vi "AttackerBallOutOfFieldSkill.vi"(6 "DistanceToBallOut":i32, 8 "error in (no error)":errorcluster, 9 "Game":refnum<class "Game.lvclass">, 10 "Robot":refnum<class "Robot.lvclass">, 11 "AttackerBallOutOfFieldSkill in":refnum<class "AttackerBallOutOfFieldSkill.lvclass">) -> (0 "error out":errorcluster, 2 "Robot out":refnum<class "Robot.lvclass">, 3 "AttackerBallOutOfFieldSkill out":refnum<class "AttackerBallOutOfFieldSkill.lvclass">)   [LabVIEW 2018, in "AttackerBallOutOfFieldSkill.lvclass"]
uses:
  AttackerBallOutOfFieldSkill.lvclass
  Game_class/Game.lvclass
  Robot_class/Robot.lvclass
  C:/Users/Gustavo/Desktop/RoboIME/SimplePass/SSL_AI/Object_class/Object.lvclass
  Object_class/Object.lvclass/Object.ctl
  Game_class/Game.lvclass/Game.ctl
  Robot_class/Robot.lvclass/Robot.ctl
  Game_class/Read BallRef.vi
  Game_class/Read FieldRef.vi
  Object_class/Read x.vi
  Object_class/Read y.vi
  Robot_class/Write dest_x.vi
  Robot_class/Write dest_y.vi
  Robot_class/Write dest_orientation.vi
  Ball_class/Ball.lvclass
  Field_class/Field.lvclass
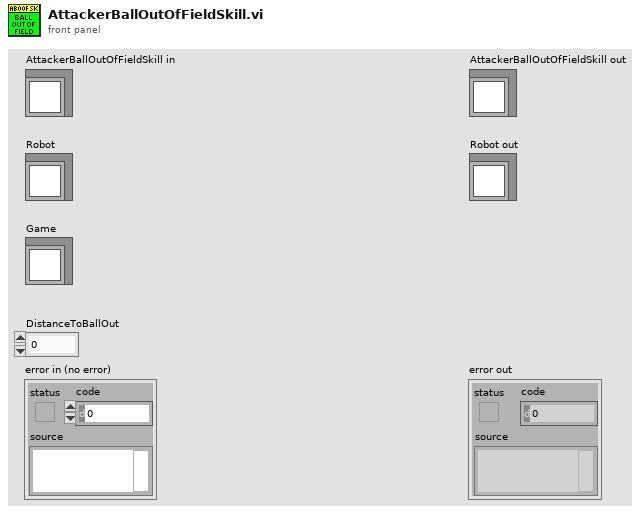
[diagram p1: front panel]
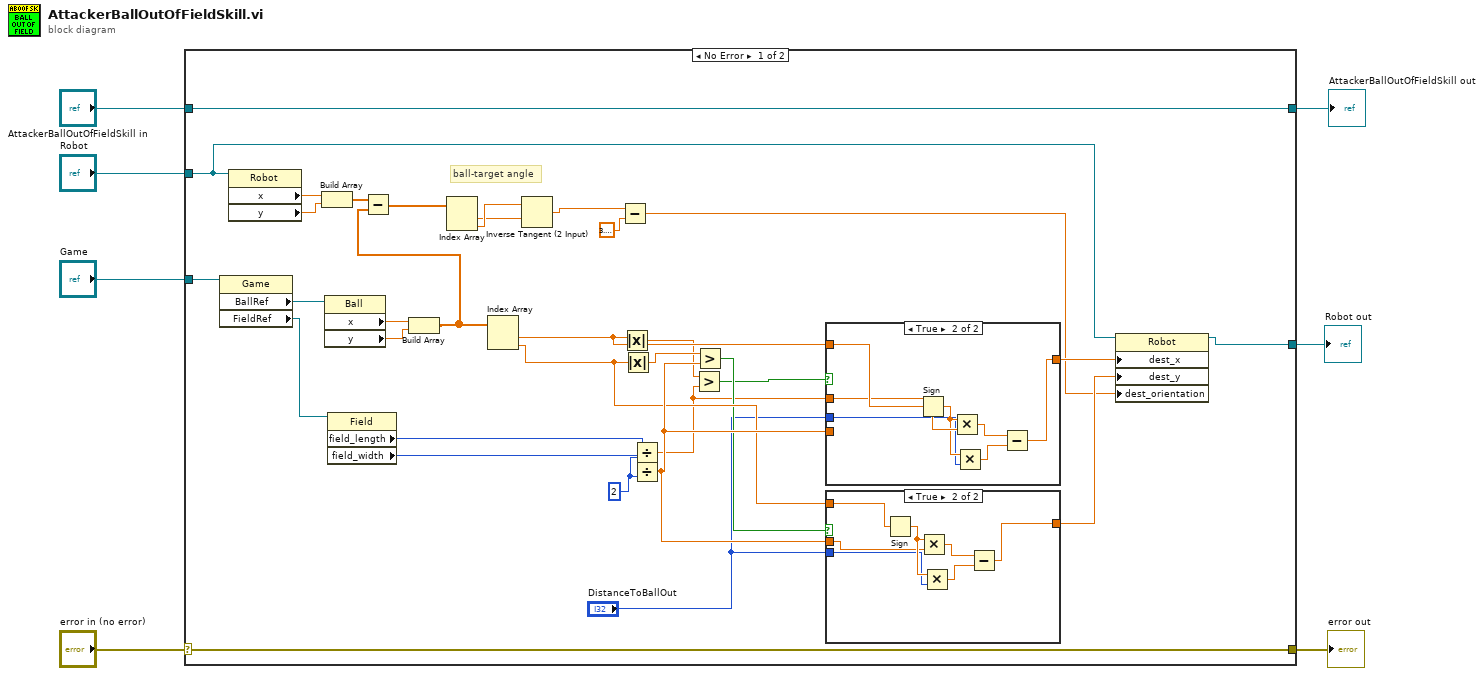
[diagram p0: block diagram]
diagram:
  n1 = case shown="No Error" "error in (no error)" {
    selector: "error in (no error)" -> [w39 w59]
    tunnel: [w39 w59] -> w6
    tunnel: [w40 w58] -> w4
    tunnel: "AttackerBallOutOfFieldSkill in" -> [w40 w58]
    tunnel: "Robot" -> [w13 w57]
    tunnel: "Game" -> [w12 _]
    tunnel: [w11 w57] -> w1
    frame No Error {
      w27 = u32 2 ("y")
      # "ball-target angle"
      n2 = property class="Game"(reference=w12) -> ("BallRef"=w23:refnum<class "Ball.lvclass">, "FieldRef"=w19:refnum<class "Field.lvclass">)  [unwired: 1 in, 2 out]
      n3 = property class="Robot"(reference=w13) -> ("x"=w26:dbl, "y"=w25:dbl)  [unwired: 1 in, 2 out]
      n4 = Build Array(w26, w25) -> (w24:dbl[])
      n5 = property class="Ball"(reference=w23) -> ("x"=w22:dbl, "y"=w21:dbl)  [unwired: 1 in, 2 out]
      n6 = property class="Field"(reference=w19) -> ("field_length"=w18:i32, "field_width"=w17:i32)  [unwired: 1 in, 2 out]
      n7 = Build Array(w22, w21) -> (w20:dbl[])
      n8 = Subtract(x=w24, y=w20) -> (x-y=w34:dbl[])
      n9 = Index Array(array=w34) -> (element #1=w32:dbl, element #2=w33:dbl)  [unwired: 2 in]
      n10 = Index Array(array=w20) -> (element #1=w31:dbl, element #2=w37:dbl)  [unwired: 2 in]
      n11 = Inverse Tangent (2 Input)(1:w32, 2:w33) -> (0:w10:dbl)
      n12 = Subtract(x=w10, y=3.141592653589793) -> (x-y=w8:dbl)
      n13 = Absolute Value(x=w31) -> (abs(x)=w28:dbl)
      n14 = Absolute Value(x=w37) -> (abs(x)=w30:dbl)
      n15 = Divide(x=w18, y=w27) -> (x/y=w35:dbl)
      n16 = Divide(x=w17, y=w27) -> (x/y=w38:dbl)
      n17 = Greater?(x=w28, y=w35) -> (0:w29:bool)
      n18 = Greater?(x=w30, y=w38) -> (0:w36:bool)
      n19 = case shown="True" w29 {
        tunnel: w31 -> [w49 w56]
        tunnel: [w49 w54] -> w15
        tunnel: w35 -> [_ w55]
        tunnel: w38 -> [_ _]
        tunnel: "DistanceToBallOut" -> [_ w50]
        frame False {
        }
        frame True {
          n20 = Sign(1:w56) -> (0:w52:dbl)
          n21 = Multiply(x=w52, y=w55) -> (x*y=w53:dbl)
          n22 = Multiply(x=w52, y=w50) -> (x*y=w51:dbl)
          n23 = Subtract(x=w53, y=w51) -> (x-y=w54:dbl)
        }
      }
      n24 = case shown="True" w36 {
        tunnel: w37 -> [w41 w45]
        tunnel: w38 -> [_ w43]
        tunnel: [w41 w44] -> w14
        tunnel: "DistanceToBallOut" -> [_ w42]
        frame False {
        }
        frame True {
          n25 = Sign(1:w45) -> (0:w47:dbl)
          n26 = Multiply(x=w47, y=w43) -> (x*y=w48:dbl)
          n27 = Multiply(x=w47, y=w42) -> (x*y=w46:dbl)
          n28 = Subtract(x=w48, y=w46) -> (x-y=w44:dbl)
        }
      }
      n29 = property class="Robot"(reference=w13, "dest_x"=w15, "dest_y"=w14, "dest_orientation"=w8) -> (reference out=w11:refnum<class "Robot.lvclass">)  [unwired: 1 in, 1 out]
    }
    frame Error {
    }
  }
  "error out" <- w6
  "AttackerBallOutOfFieldSkill out" <- w4
  "Robot out" <- w1
